vi "GVZwangsMPVPos.vi"() -> ()   [LabVIEW 2010]
panel:
  out "ZwangsMPV!":i32
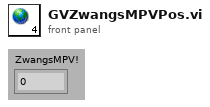
[diagram p1: front panel]
diagram:
